vi "Read.vi"(8 "ErrorIn":errorcluster, 11 "VISAIn":refnum<visa-resource-name>) -> (0 "ErrorOut":errorcluster, 2 "Data":string, 3 "VISAOut":refnum<visa-resource-name>)   [LabVIEW 2017, in "I28Drivers.lvlib"]
uses:
  I28Drivers.lvlib
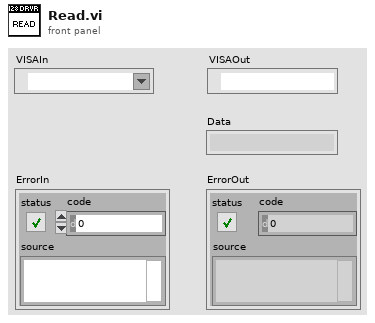
[diagram p1: front panel]
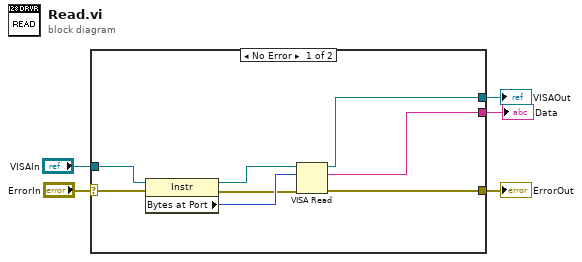
[diagram p0: block diagram]
diagram:
  n1 = case shown="No Error" "ErrorIn" {
    selector: "ErrorIn" -> [w13 w14]
    tunnel: [w7 w14] -> w4
    tunnel: "VISAIn" -> [w12 w15]
    tunnel: [w8 w15] -> w2
    tunnel: [w6 _] -> w1
    frame No Error {
      n2 = property class="Instr"(reference=w12, error in=w13) -> (reference out=w11:refnum<visa-resource-name>, error out=w9:errorcluster, "Bytes at Port"=w10:u32)
      n3 = VISA Read(VISA resource name=w11, byte count=w10, error in (no error)=w9) -> (VISA resource name out=w8:refnum<visa-resource-name>, read buffer=w6:string, error out=w7:errorcluster)  [unwired: 1 out]
    }
    frame Error {
    }
  }
  "ErrorOut" <- w4
  "VISAOut" <- w2
  "Data" <- w1
